vi "gl_XYZStage globals.vi"() -> ()   [LabVIEW 2020]
panel:
  out "Motor E-stop":bool
  out "XYZ stage initialised":bool
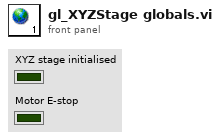
[diagram p1: front panel]
diagram:
